vi "Read State.vi"(8 "error in (no error)":errorcluster, 11 "TCP_Streamer_Subscriber in":refnum<class "TCP_Streamer_Subscriber.lvclass">) -> (0 "error out":errorcluster, 2 "State":T1, 3 "TCP_Streamer_Subscriber out":refnum<class "TCP_Streamer_Subscriber.lvclass">)   [LabVIEW 2021, in "TCP_Streamer_Subscriber.lvclass"]
uses:
  TCP_Streamer_Subscriber.lvclass
  TCP_Streamer_Subscriber.lvclass/TCP_Streamer_Subscriber.ctl
  Typedef/State.ctl
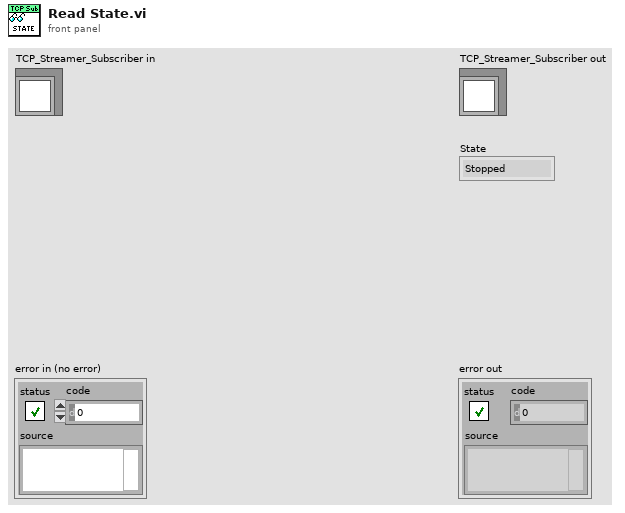
[diagram p1: front panel]
types:
  T1 = typedef "TCP_Streamer_Subscriber.lvclass/State.ctl" = enum16{"Stopped", "Connecting", "Receiving"}
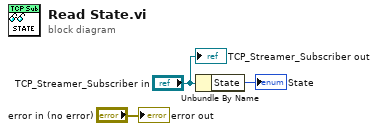
[diagram p0: block diagram]
diagram:
  n1 = Unbundle By Name("TCP_Streamer_Subscriber in") -> ("State"=→"State":T1)
  "error out" <- "error in (no error)"
  "TCP_Streamer_Subscriber out" <- "TCP_Streamer_Subscriber in"
